vi "SPI Set Bit Order.vi"(8 "Error In":errorcluster, 9 "SPI Bit Order":T1, 10 "SPI Channel":u8, 11 "LINX Device Config":T2) -> (0 "Error Out":errorcluster, 3 "LINX Device Config":T2)   [LabVIEW 2014, in "LMH-LINX.lvlib" / "Device.lvlib"]
doc: "Set the bit order of the specified SPI Channel."
uses:
  <vilib>/MakerHub/LINX/Private/Device/Device.lvlib
  <vilib>/MakerHub/LINX/Private/Device/Type Defs/LINX Device Config.ctl
  <vilib>/MakerHub/LINX/Private/Type Defs/Interface.ctl
  <vilib>/MakerHub/LINX/Private/Device/Type Defs/TCP Config.ctl
  <vilib>/MakerHub/LINX/Private/Device/Type Defs/Channels.ctl
  <vilib>/MakerHub/LINX/Private/Type Defs/Peripherals/SPI/SPI Bit Order.ctl
  <vilib>/MakerHub/LINX/Private/Type Defs/Error Type.ctl
  <vilib>/MakerHub/LINX/LMH-LINX.lvlib
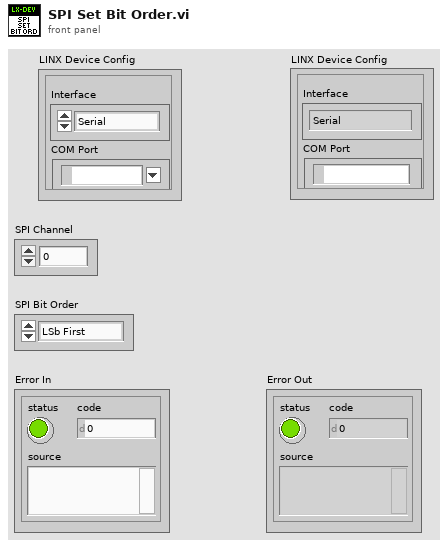
[diagram p1: front panel]
types:
  T1 = typedef "LMH-LINX.lvlib/SPI Bit Order.ctl" = enum8{"LSb First", "MSb First"}
  T2 = typedef "LMH-LINX.lvlib/Device.lvlib/LINX Device Config.ctl" = cluster{"Interface":T3, "COM Port":refnum<visa-resource-name>, "TCP Configuration":T4, "Device Family":u8, "Device ID":u8, "Device Name":string, "TCP Ref":refnum<k5>, "Channels":T5}
  T3 = typedef "LMH-LINX.lvlib/Interface.ctl" = enum16{"Serial", "TCP"}
  T4 = typedef "LMH-LINX.lvlib/Device.lvlib/TCP Config.ctl" = cluster{"IP Address":string, "Port":u16}
  T5 = typedef "LMH-LINX.lvlib/Channels.ctl" = cluster{"DI":u8[], "DO":u8[], "AI":u8[], "AO":u8[], "PWM":u8[], "QE":u8[], "UART":u8[], "I2C 2":u8[], "SPI":u8[], "CAN":u8[], "Servo":u8[], "AI Ref (V)":dbl, "AI Resolution (Bits)":u8, "AO Ref (V)":dbl, "AO Resolution (Bits)":u8}
  T6 = typedef "LMH-LINX.lvlib/Error Type.ctl" = enum16{"Unknown", "Timeout", "Corrupt Return Packet", "Unable To Connect", "Command Not Supported", "Channel DNE", "Invalid COM Config", "Firmware Version Mismatch", "myRIO Support", "CMD Specific Error", "Local IO Not Supported"}
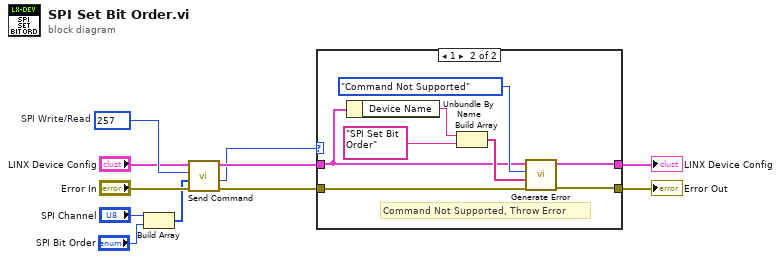
[diagram p0: block diagram]
diagram:
  w10 = u16 257  # SPI Write/Read
  n1 = Build Array("SPI Channel", "SPI Bit Order") -> (w3:u8[])
  n2 = call <vilib>:"Send Command.vi"("Error In"="Error In", "ARGS"=w3, "CMD"=w10, "LINX Device Config"="LINX Device Config") -> ("Error Out"=w5:errorcluster, "Status"=w1:u8, "LINX Device Config"=w7:T2)  [unwired: 4 in, 1 out]
  n3 = case shown="1" w1 {
    tunnel: [w13 w19] -> w8
    tunnel: w7 -> [w13 w15]
    tunnel: [w12 w20] -> w6
    tunnel: w5 -> [w12 w21]
    frame 0, Default {
      # "Status OK, Process Data"
    }
    frame 1 {
      # "Command Not Supported, Throw Error"
      n4 = Unbundle By Name(w15) -> ("Device Name"=w14:string)
      n5 = Build Array(w14, "SPI Set Bit Order") -> (w16:string[])
      n6 = call <vilib>:"Generate Error.vi"("Error In"=w21, "Arguments"=w16, "Error Type"=Error_Type."Command Not Supported", "LINX Device Config"=w15) -> ("Error Out"=w20:errorcluster, "Dup LINX Device Config"=w19:T2)  [unwired: 6 in]
    }
  }
  "Error Out" <- w6
  "LINX Device Config" <- w8
